vi "Add Topic Subscriber.vi"(8 "error in (no error)":errorcluster, 9 "Subscriber Transport":refnum<class "ITransport.lvclass">, 10 "Subscriber Name":string, 11 "Topic in":refnum<class "Topic.lvclass">) -> (0 "error out":errorcluster, 3 "Topic out":refnum<class "Topic.lvclass">)   [LabVIEW 2015, in "Mediator.lvlib" / "Topic.lvclass"]
uses:
  Topic.lvclass
  Transport/ITransport/ITransport.lvclass
  Topic.lvclass/Topic.ctl
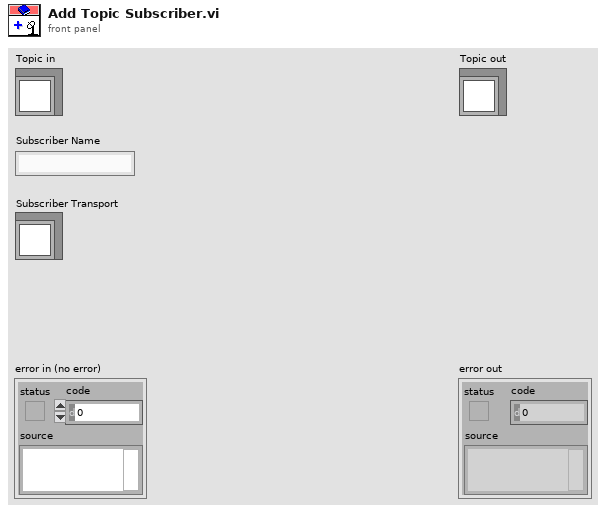
[diagram p1: front panel]
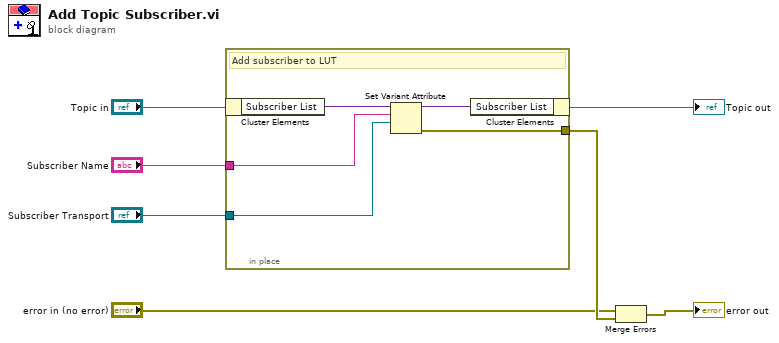
[diagram p0: block diagram]
diagram:
  n1 = in-place {
    in-place-border: [w10] -> w7
    in-place-border: "Subscriber Name" -> [w9]
    in-place-border: "Subscriber Transport" -> [w8]
    # "Add subscriber to LUT"
    n2 = in-place-cluster #1("Topic in") -> ("Subscriber List"=w12:variant)
    n3 = Set Variant Attribute(Variant=w12, name=w9, value=w8) -> (Variant out=w11:variant, error out=w10:errorcluster)  [unwired: 1 in, 1 out]
    n4 = in-place-cluster #1("Subscriber List"=w11) -> (→"Topic out":refnum<class "Topic.lvclass">)
  }
  n5 = Merge Errors("error in (no error)", w7) -> (→"error out":errorcluster)
